vi "FL_Decode_RAW_to_DEC_last_out.vi"(3 "Input array of timestamps":timestamp[](array[timestamp]), 6 "Sensor board size":string="Small", 7 "read buffer":string) -> (0 "Output timestamp":timestamp, 1 "DEC output":sgl[](array[numeric]))   [LabVIEW 2018, in "Tracker.lvlib"]
uses:
  Tracker.lvlib
panel:
  out "offset past match":i32
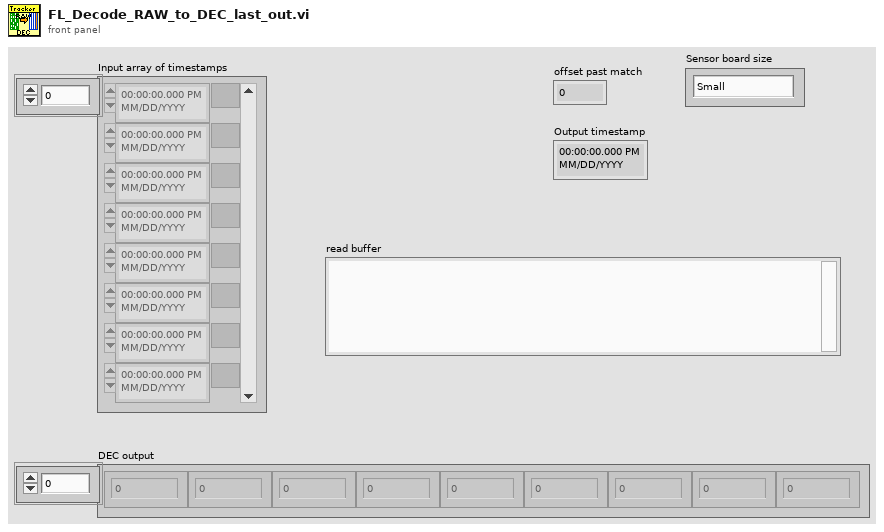
[diagram p1: front panel]
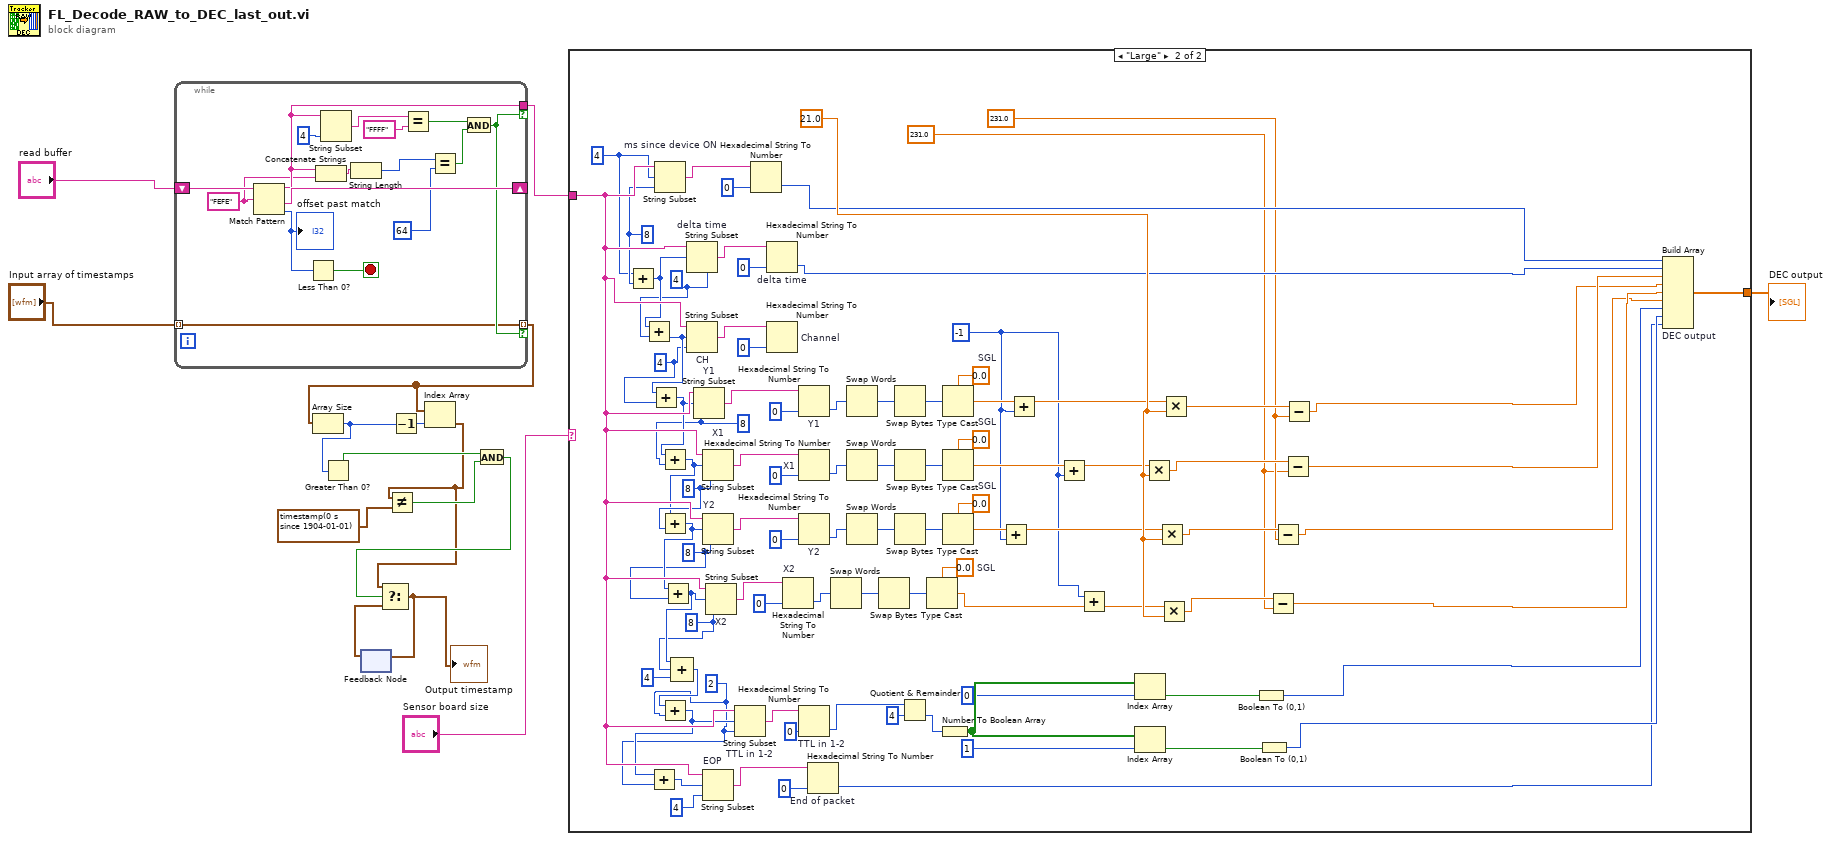
[diagram p0: block diagram]
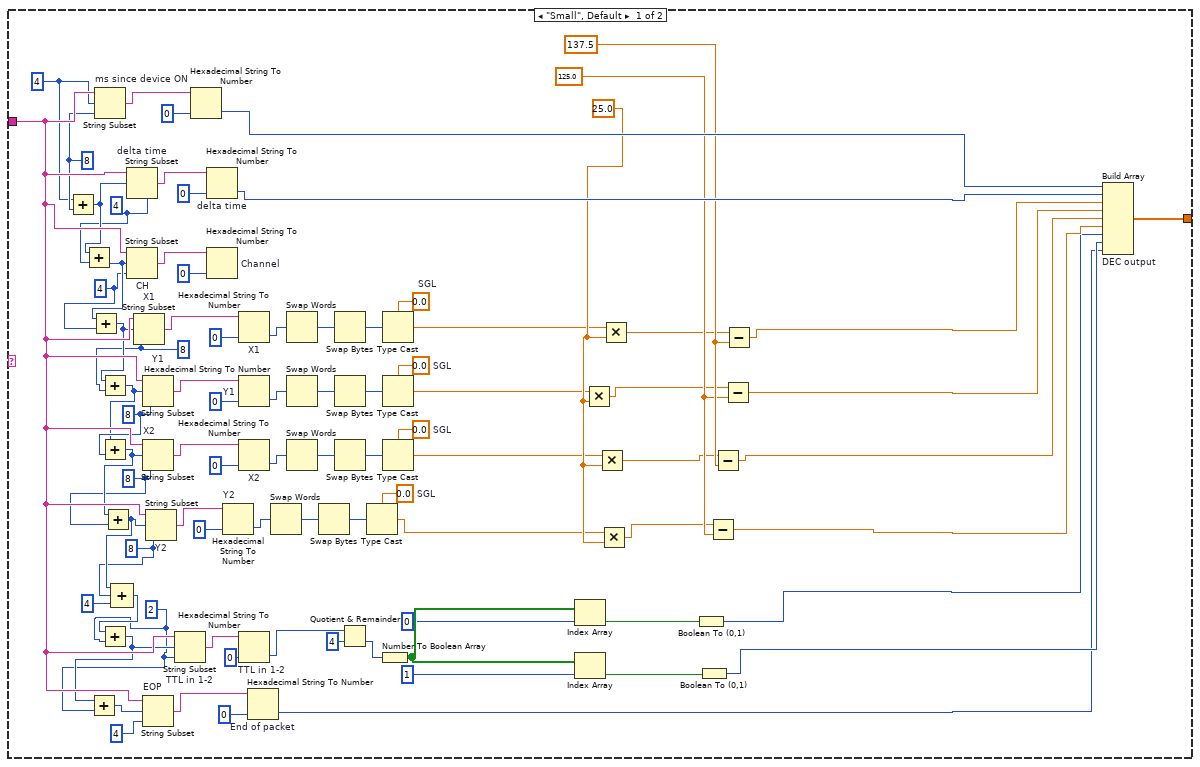
[diagram p2: hidden frame]
diagram:
  n1 = while {
    shift-right: [w30] -> _
    shift-left: "read buffer" -> [w31]
    tunnel: [w20] -> w14 if=w17
    tunnel: [w16] -> w10 mode=indexing if=w17
    tunnel: "Input array of timestamps" -> [w16] mode=indexing
    stop <- w28 stop-if-true
    w18 = "FEFE" ("regular expression")
    n2 = Match Pattern(string=w31, regular expression=w18) -> (before substring=w20:string, after substring=w30:string, offset past match=w29:i32)  [unwired: 1 in, 1 out]
    "offset past match" <- w29
    n3 = Less Than 0?(x=w29) -> (x < 0?=w28:bool)
    n4 = Concatenate Strings(w20, w18) -> (w19:string)
    n5 = String Subset(string=w20, length (rest)=4 ("length (rest)")) -> (substring=w26:string)  [unwired: 1 in]
    n6 = String Length(string=w19) -> (length=w24:i32)
    n7 = Equal?(x=w26, y="FFFF") -> (x = y?=w22:bool)
    n8 = Equal?(x=w24, y=64) -> (x = y?=w21:bool)
    n9 = And(x=w22, y=w21) -> (x .and. y?=w17:bool)
  }
  n10 = Array Size(array=w10) -> (size(s)=w8:i32)
  n11 = Greater Than 0?(x=w8) -> (x > 0?=w6:bool)
  n12 = feedback #1() -> (w1:timestamp)  [unwired: 1 in]
  n13 = Decrement(x=w8) -> (x-1=w9:i32)
  n14 = Index Array(array=w10, index=w9) -> (element=w3:timestamp)
  n15 = Not Equal?(x=w3, y=timestamp(0 s since 1904-01-01)) -> (x != y?=w5:bool)
  n16 = And(x=w6, y=w5) -> (x .and. y?=w4:bool)
  n17 = Select(t=w3, s=w4, f=w1) -> (s? t:f=w2:timestamp)
  "Output timestamp" <- w2
  n18 = feedback-in #1(w2) -> ()
  n19 = case shown="\"Large\"" "Sensor board size" {
    tunnel: w14 -> [w115 w204]
    tunnel: [w114 w203] -> w13
    frame "Small", Default {
      w42 = sgl 137.5 ("Half-width of the sensor board")
      w41 = sgl 125.0 ("Half-height of the sensor board")
      w36 = sgl 25.0 ("Sensors grid step")
      w43 = 4
      w53 = 2 ("length (rest)")
      w64 = sgl 0.0  # SGL
      w70 = sgl 0.0  # SGL
      w76 = sgl 0.0  # SGL
      w81 = sgl 0.0  # SGL
      w58 = 8 ("length (rest)")
      w94 = 8 ("length (rest)")
      w97 = 8 ("length (rest)")
      w98 = 8 ("length (rest)")
      w100 = 4 ("length (rest)")
      w102 = 4 ("length (rest)")
      w104 = 8 ("length (rest)")
      n20 = Add(x=w43, y=w104) -> (x+y=w103:i32)
      n21 = Add(x=w103, y=w102) -> (x+y=w101:i32)
      n22 = Add(x=w101, y=w100) -> (x+y=w99:i32)
      n23 = String Subset "ms since device ON"(string=w115, offset (0)=w43, length (rest)=w104) -> (substring=w91:string)
      n24 = Add(x=w99, y=w98) -> (x+y=w96:i32)
      n25 = Add(x=w96, y=w97) -> (x+y=w95:i32)
      n26 = Add(x=w95, y=w94) -> (x+y=w59:i32)
      n27 = Compound Arithmetic op=unknown(w59, w58, 4 ("value")) -> (w55:i32)
      n28 = Add(x=w55, y=w53) -> (x+y=w54:i32)
      n29 = Add(x=w54, y=w53) -> (x+y=w93:i32)
      n30 = String Subset "delta time"(string=w115, offset (0)=w103, length (rest)=w102) -> (substring=w88:string)
      n31 = String Subset "CH"(string=w115, offset (0)=w101, length (rest)=w100) -> (substring=w86:string)
      n32 = String Subset "X1"(string=w115, offset (0)=w99, length (rest)=w98) -> (substring=w85:string)
      n33 = String Subset "Y1"(string=w115, offset (0)=w96, length (rest)=w97) -> (substring=w74:string)
      n34 = String Subset "X2"(string=w115, offset (0)=w95, length (rest)=w94) -> (substring=w68:string)
      n35 = String Subset "EOP"(string=w115, offset (0)=w93, length (rest)=4 ("length (rest)")) -> (substring=w60:string)
      n36 = String Subset "Y2"(string=w115, offset (0)=w59, length (rest)=w58) -> (substring=w62:string)
      n37 = String Subset "TTL in 1-2"(string=w115, offset (0)=w54, length (rest)=w53) -> (substring=w57:string)
      n38 = Hexadecimal String To Number ("ms since ON")(string=w91, default (0uL)=u32 0 ("default (0 U32)")) -> (number=w113:u32)  [unwired: 1 in, 1 out]
      n39 = Hexadecimal String To Number "delta time"(string=w88, default (0uL)=u32 0 ("default (0 U32)")) -> (number=w112:u32)  [unwired: 1 in, 1 out]
      n40 = Hexadecimal String To Number "Channel"(string=w86, default (0uL)=u32 0 ("default (0 U32)")) -> ()  [unwired: 1 in, 2 out]
      n41 = Hexadecimal String To Number "Y2"(string=w62, default (0uL)=u32 0 ("default (0 U32)")) -> (number=w66:u32)  [unwired: 1 in, 1 out]
      n42 = Hexadecimal String To Number "X1"(string=w85, default (0uL)=u32 0 ("default (0 U32)")) -> (number=w83:u32)  [unwired: 1 in, 1 out]
      n43 = Hexadecimal String To Number "Y1"(string=w74, default (0uL)=u32 0 ("default (0 U32)")) -> (number=w78:u32)  [unwired: 1 in, 1 out]
      n44 = Hexadecimal String To Number "X2"(string=w68, default (0uL)=u32 0 ("default (0 U32)")) -> (number=w72:u32)  [unwired: 1 in, 1 out]
      n45 = Hexadecimal String To Number "TTL in 1-2"(string=w57, default (0uL)=u32 0 ("default (0 U32)")) -> (number=w50:u32)  [unwired: 1 in, 1 out]
      n46 = Hexadecimal String To Number "End of packet"(string=w60, default (0uL)=u32 0 ("default (0 U32)")) -> (number=w105:u32)  [unwired: 1 in, 1 out]
      n47 = Swap Words(1:w66) -> (0:w65:u32)
      n48 = Swap Words(1:w83) -> (0:w82:u32)
      n49 = Swap Words(1:w78) -> (0:w77:u32)
      n50 = Swap Words(1:w72) -> (0:w71:u32)
      n51 = Swap Bytes(anything=w65) -> (byte swapped=w63:u32)
      n52 = Swap Bytes(anything=w82) -> (byte swapped=w80:u32)
      n53 = Swap Bytes(anything=w77) -> (byte swapped=w75:u32)
      n54 = Swap Bytes(anything=w71) -> (byte swapped=w69:u32)
      n55 = Quotient & Remainder(x=w50, y=u32 4) -> (floor(x/y)=w49:u32)  [unwired: 1 out]
      n56 = Type Cast(type=w64, x=w63) -> (*(type *) &x=w32:sgl)
      n57 = Number To Boolean Array(number=w49) -> (Boolean array=w48:bool[])
      n58 = Type Cast(type=w81, x=w80) -> (*(type *) &x=w35:sgl)
      n59 = Type Cast(type=w76, x=w75) -> (*(type *) &x=w34:sgl)
      n60 = Type Cast(type=w70, x=w69) -> (*(type *) &x=w33:sgl)
      n61 = Index Array(array=w48, index=0) -> (element=w45:bool)
      n62 = Index Array(array=w48, index=1) -> (element=w44:bool)
      n63 = Multiply(x=w34, y=w36) -> (x*y=w39:sgl)
      n64 = Multiply(x=w33, y=w36) -> (x*y=w38:sgl)
      n65 = Multiply(x=w32, y=w36) -> (x*y=w37:sgl)
      n66 = Multiply(x=w35, y=w36) -> (x*y=w40:sgl)
      n67 = Boolean To (0,1)(Boolean=w45) -> (0, 1=w107:i16)
      n68 = Boolean To (0,1)(Boolean=w44) -> (0, 1=w106:i16)
      n69 = Subtract(x=w37, y=w41) -> (x-y=w108:sgl)
      n70 = Subtract(x=w38, y=w42) -> (x-y=w109:sgl)
      n71 = Subtract(x=w39, y=w41) -> (x-y=w110:sgl)
      n72 = Subtract(x=w40, y=w42) -> (x-y=w111:sgl)
      n73 = Build Array "DEC output"(w113, w112, w111, w110, w109, w108, w107, w106, w105) -> (w114:sgl[])
    }
    frame "Large" {
      w116 = -1
      w126 = sgl 231.0 ("Half-width of the sensor board")
      w125 = sgl 231.0 ("Half-height of the sensor board")
      w202 = sgl 21.0 ("Sensors grid step")
      w127 = 4
      w137 = 2 ("length (rest)")
      w153 = sgl 0.0  # SGL
      w160 = sgl 0.0  # SGL
      w167 = sgl 0.0  # SGL
      w173 = sgl 0.0  # SGL
      w142 = 8 ("length (rest)")
      w186 = 8 ("length (rest)")
      w189 = 8 ("length (rest)")
      w190 = 8 ("length (rest)")
      w192 = 4 ("length (rest)")
      w194 = 4 ("length (rest)")
      w196 = 8 ("length (rest)")
      n74 = Add(x=w127, y=w196) -> (x+y=w195:i32)
      n75 = Add(x=w195, y=w194) -> (x+y=w193:i32)
      n76 = Add(x=w193, y=w192) -> (x+y=w191:i32)
      n77 = String Subset "ms since device ON"(string=w204, offset (0)=w127, length (rest)=w196) -> (substring=w183:string)
      n78 = Add(x=w191, y=w190) -> (x+y=w188:i32)
      n79 = Add(x=w188, y=w189) -> (x+y=w187:i32)
      n80 = Add(x=w187, y=w186) -> (x+y=w143:i32)
      n81 = Compound Arithmetic op=unknown(w143, w142, 4 ("value")) -> (w139:i32)
      n82 = Add(x=w139, y=w137) -> (x+y=w138:i32)
      n83 = Add(x=w138, y=w137) -> (x+y=w185:i32)
      n84 = String Subset "delta time"(string=w204, offset (0)=w195, length (rest)=w194) -> (substring=w180:string)
      n85 = String Subset "CH"(string=w204, offset (0)=w193, length (rest)=w192) -> (substring=w178:string)
      n86 = String Subset "Y1"(string=w204, offset (0)=w191, length (rest)=w190) -> (substring=w177:string)
      n87 = String Subset "X1"(string=w204, offset (0)=w188, length (rest)=w189) -> (substring=w165:string)
      n88 = String Subset "Y2"(string=w204, offset (0)=w187, length (rest)=w186) -> (substring=w158:string)
      n89 = String Subset "EOP"(string=w204, offset (0)=w185, length (rest)=4 ("length (rest)")) -> (substring=w148:string)
      n90 = String Subset "X2"(string=w204, offset (0)=w143, length (rest)=w142) -> (substring=w151:string)
      n91 = String Subset "TTL in 1-2"(string=w204, offset (0)=w138, length (rest)=w137) -> (substring=w141:string)
      n92 = Hexadecimal String To Number ("ms since ON")(string=w183, default (0uL)=u32 0 ("default (0 U32)")) -> (number=w201:u32)  [unwired: 1 in, 1 out]
      n93 = Hexadecimal String To Number "delta time"(string=w180, default (0uL)=u32 0 ("default (0 U32)")) -> (number=w200:u32)  [unwired: 1 in, 1 out]
      n94 = Hexadecimal String To Number "Channel"(string=w178, default (0uL)=u32 0 ("default (0 U32)")) -> ()  [unwired: 1 in, 2 out]
      n95 = Hexadecimal String To Number "X2"(string=w151, default (0uL)=u32 0 ("default (0 U32)")) -> (number=w155:u32)  [unwired: 1 in, 1 out]
      n96 = Hexadecimal String To Number "Y1"(string=w177, default (0uL)=u32 0 ("default (0 U32)")) -> (number=w175:u32)  [unwired: 1 in, 1 out]
      n97 = Hexadecimal String To Number "X1"(string=w165, default (0uL)=u32 0 ("default (0 U32)")) -> (number=w169:u32)  [unwired: 1 in, 1 out]
      n98 = Hexadecimal String To Number "Y2"(string=w158, default (0uL)=u32 0 ("default (0 U32)")) -> (number=w162:u32)  [unwired: 1 in, 1 out]
      n99 = Hexadecimal String To Number "TTL in 1-2"(string=w141, default (0uL)=u32 0 ("default (0 U32)")) -> (number=w134:u32)  [unwired: 1 in, 1 out]
      n100 = Hexadecimal String To Number "End of packet"(string=w148, default (0uL)=u32 0 ("default (0 U32)")) -> (number=w197:u32)  [unwired: 1 in, 1 out]
      n101 = Swap Words(1:w155) -> (0:w154:u32)
      n102 = Swap Words(1:w175) -> (0:w174:u32)
      n103 = Swap Words(1:w169) -> (0:w168:u32)
      n104 = Swap Words(1:w162) -> (0:w161:u32)
      n105 = Swap Bytes(anything=w154) -> (byte swapped=w152:u32)
      n106 = Swap Bytes(anything=w174) -> (byte swapped=w172:u32)
      n107 = Swap Bytes(anything=w168) -> (byte swapped=w166:u32)
      n108 = Swap Bytes(anything=w161) -> (byte swapped=w159:u32)
      n109 = Quotient & Remainder(x=w134, y=u32 4) -> (floor(x/y)=w133:u32)  [unwired: 1 out]
      n110 = Type Cast(type=w153, x=w152) -> (*(type *) &x=w150:sgl)
      n111 = Number To Boolean Array(number=w133) -> (Boolean array=w132:bool[])
      n112 = Type Cast(type=w173, x=w172) -> (*(type *) &x=w171:sgl)
      n113 = Type Cast(type=w167, x=w166) -> (*(type *) &x=w164:sgl)
      n114 = Type Cast(type=w160, x=w159) -> (*(type *) &x=w157:sgl)
      n115 = Add(x=w157, y=w116) -> (x+y=w118:sgl)
      n116 = Add(x=w171, y=w116) -> (x+y=w120:sgl)
      n117 = Add(x=w164, y=w116) -> (x+y=w119:sgl)
      n118 = Add(x=w116, y=w150) -> (x+y=w117:sgl)
      n119 = Index Array(array=w132, index=0) -> (element=w129:bool)
      n120 = Index Array(array=w132, index=1) -> (element=w128:bool)
      n121 = Multiply(x=w119, y=w202) -> (x*y=w145:sgl)
      n122 = Multiply(x=w118, y=w202) -> (x*y=w146:sgl)
      n123 = Multiply(x=w117, y=w202) -> (x*y=w144:sgl)
      n124 = Multiply(x=w120, y=w202) -> (x*y=w147:sgl)
      n125 = Boolean To (0,1)(Boolean=w129) -> (0, 1=w199:i16)
      n126 = Boolean To (0,1)(Boolean=w128) -> (0, 1=w198:i16)
      n127 = Subtract(x=w144, y=w125) -> (x-y=w122:sgl)
      n128 = Subtract(x=w146, y=w126) -> (x-y=w121:sgl)
      n129 = Subtract(x=w145, y=w125) -> (x-y=w124:sgl)
      n130 = Subtract(x=w147, y=w126) -> (x-y=w123:sgl)
      n131 = Build Array "DEC output"(w201, w200, w124, w123, w122, w121, w199, w198, w197) -> (w203:sgl[])
    }
  }
  "DEC output" <- w13
